vi "dfd_Maxflat Filter Design Generate Poly for M_NotZero.vi"(9 "M":i32=1, 10 "N":i32=2, 11 "L":i32=3) -> (0 "truncated APT":dbl[](array[numeric]), 1 "truncated APR-APT":dbl[](array[numeric]), 2 "APT":dbl[](array[numeric]), 3 "APR-APT":dbl[](array[numeric]))   [LabVIEW 2017, in "NI_DigFilter_Design.lvlib"]
doc: "Generates the polynomial for M!=0."
uses:
  <vilib>/addons/Digital Filter Design/NI_DigFilter_Design.lvlib
  <vilib>/addons/Digital Filter Design/NI_DigFilter_Process.lvlib
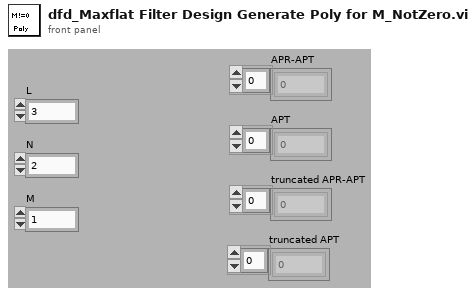
[diagram p1: front panel]
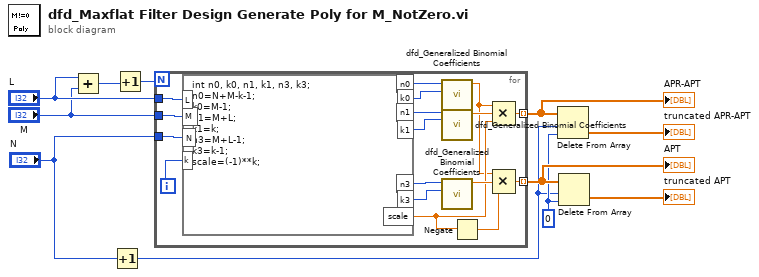
[diagram p0: block diagram]
diagram:
  w7 = 0
  n1 = Add(x="L", y="M") -> (x+y=w2:i32)
  n2 = Increment(x="N") -> (x+1=w5:i32)
  n3 = Increment(x=w2) -> (x+1=w1:i32)
  n4 = for {
    N: w1 -> [_]
    tunnel: "L" -> [w28]
    tunnel: "M" -> [w27]
    tunnel: "N" -> [w26]
    tunnel: [w17] -> w10 mode=indexing
    tunnel: [w15] -> w11 mode=indexing
    i -> [w25]
    n5 = formula code="int n0, k0, n1, k1, n3, k3;\nn0=N+M-k-1;\nk0=M-1;\nn1=M+L;\nk1=k;\nn3=M+L-1;\nk3=k-1;\nscale=(-1)**k;"("N"=w26, "M"=w27, "k"=w25, "L"=w28) -> ("n0"=w24:i32, "k0"=w23:i32, "n1"=w22:i32, "k1"=w21:i32, "n3"=w20:i32, "k3"=w19:i32, "scale"=w14:dbl)
    n6 = call <vilib>:"dfd_Generalized Binomial Coefficients.vi"("k"=w23, "n"=w24) -> ("binomial coefficient (n,k)"=w12:dbl)  [unwired: 1 in, 8 out]
    n7 = call <vilib>:"dfd_Generalized Binomial Coefficients.vi"("k"=w21, "n"=w22) -> ("binomial coefficient (n,k)"=w18:dbl)  [unwired: 1 in, 8 out]
    n8 = call <vilib>:"dfd_Generalized Binomial Coefficients.vi"("k"=w19, "n"=w20) -> ("binomial coefficient (n,k)"=w16:dbl)  [unwired: 1 in, 8 out]
    n9 = Negate(x=w14) -> (-x=w13:dbl)
    n10 = Compound Arithmetic op=MULTIPLY(w12, w18, w14) -> (w17:dbl)
    n11 = Compound Arithmetic op=MULTIPLY(w12, w16, w13) -> (w15:dbl)
  }
  "APT" <- w11
  "APR-APT" <- w10
  n12 = Delete From Array(array=w10, length=w5, index=w7) -> (deleted portion=→"truncated APR-APT":dbl[])  [unwired: 1 out]
  n13 = Delete From Array(array=w11, length=w5, index=w7) -> (deleted portion=→"truncated APT":dbl[])  [unwired: 1 out]
